vi "ACDC_Config.vi"(8 "error in (no error)":errorcluster, 9 "Input Config Array":T1[](array[typedef])=[0, 0, 0, 0, 0, 0, 0, 0, 0, 0, 0, 0, 0, 0, 0, 0, 0, 0, 0, 0, 0, 0, 0, 0, 0, 0, 0, 0, 0, 0, 0, 0] items=["AC Coupled", "DC Coupled", "IEPE AC Coupled"], 10 "Data Rate [S/s]":u32) -> (0 "error out":errorcluster)   [LabVIEW 2017, in "BOP_VibAPI_6.lvlib"]
uses:
  <vilib>/addons/InsightCM/Devices/Shared/Cms/Fpga/Acquisition/source/subVIs/VibAPI/BOP_VibAPI_6.lvlib
  <vilib>/LabVIEW Targets/FPGA/cRIO/shared/nicrio_ModuleControls/nicrio_cRIO-9232_ConfigModeRing.ctl
  <vilib>/rvi/eio/common/nirviEmuTemplatePropertySet_errors.vi
  <vilib>/eio/EIOPropertyNode/EIOPropertyNode.xnode
  <vilib>/LabVIEW Targets/FPGA/cRIO/shared/nicrio_ModuleControls/nicrio_cRIO-9232_DataRatesRing2.ctl
  <vilib>/rvi/eio/common/nirviEmuTemplatePropertyGet_errors.vi
  <vilib>/rvi/eio/common/nirviEmuTemplatePropertyGet_noerrors.vi
  <vilib>/rvi/eio/common/nirviEmuTemplatePropertySet_noerrors.vi
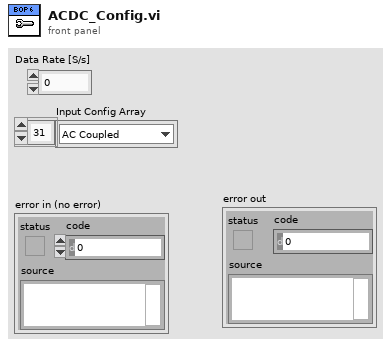
[diagram p1: front panel]
types:
  T1 = typedef "nicrio_cRIO-9232_ConfigModeRing.ctl" = u8
  T2 = typedef "nicrio_cRIO-9232_DataRatesRing2.ctl" = u8
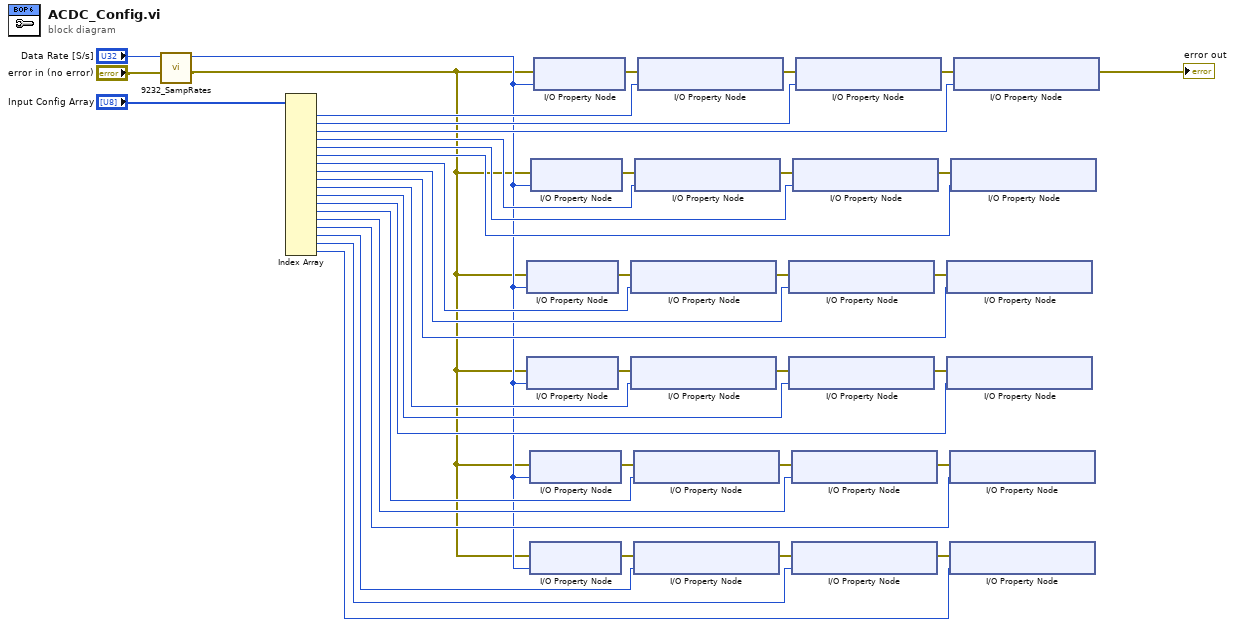
[diagram p0: block diagram]
diagram:
  n1 = call <vilib>:"9232_SampRates.vi"("error in (no error)"="error in (no error)", "Data Rate [S/s]"="Data Rate [S/s]") -> ("error out"=w3:errorcluster, "Data Rate"=w4:T2)  [unwired: 8 in]
  n2 = Index Array(array="Input Config Array") -> (element #1=w34:T1, element #2=w33:T1, element #3=w29:T1, element #4=w32:T1, element #5=w31:T1, element #6=w30:T1, element #7=w25:T1, element #8=w24:T1, element #9=w23:T1, element #10=w19:T1, element #11=w18:T1, element #12=w17:T1, element #13=w13:T1, element #14=w12:T1, element #15=w11:T1, element #16=w7:T1, element #17=w6:T1, element #18=w5:T1)  [unwired: 18 in]
  n3 = xnode "I/O Property Node"("error in"=w3, "Data Rate"=w4) -> ("error out"=w28:errorcluster)  [unwired: 1 in, 1 out]
  n4 = xnode "I/O Property Node"("error in"=w3, "Data Rate"=w4) -> ("error out"=w20:errorcluster)  [unwired: 1 in, 1 out]
  n5 = xnode "I/O Property Node"("error in"=w3, "Data Rate"=w4) -> ("error out"=w16:errorcluster)  [unwired: 1 in, 1 out]
  n6 = xnode "I/O Property Node"("error in"=w3, "Data Rate"=w4) -> ("error out"=w8:errorcluster)  [unwired: 1 in, 1 out]
  n7 = xnode "I/O Property Node"("error in"=w3, "Data Rate"=w4) -> ("error out"=w35:errorcluster)  [unwired: 1 in, 1 out]
  n8 = xnode "I/O Property Node"("error in"=w3, "Data Rate"=w4) -> ("error out"=w36:errorcluster)  [unwired: 1 in, 1 out]
  n9 = xnode "I/O Property Node"("error in"=w28, "Input Configuration"=w25) -> ("error out"=w27:errorcluster)  [unwired: 1 in, 1 out]
  n10 = xnode "I/O Property Node"("error in"=w20, "Input Configuration"=w19) -> ("error out"=w21:errorcluster)  [unwired: 1 in, 1 out]
  n11 = xnode "I/O Property Node"("error in"=w16, "Input Configuration"=w13) -> ("error out"=w15:errorcluster)  [unwired: 1 in, 1 out]
  n12 = xnode "I/O Property Node"("error in"=w8, "Input Configuration"=w7) -> ("error out"=w9:errorcluster)  [unwired: 1 in, 1 out]
  n13 = xnode "I/O Property Node"("error in"=w35, "Input Configuration"=w32) -> ("error out"=w39:errorcluster)  [unwired: 1 in, 1 out]
  n14 = xnode "I/O Property Node"("error in"=w36, "Input Configuration"=w34) -> ("error out"=w37:errorcluster)  [unwired: 1 in, 1 out]
  n15 = xnode "I/O Property Node"("error in"=w27, "Input Configuration"=w24) -> ("error out"=w26:errorcluster)  [unwired: 1 in, 1 out]
  n16 = xnode "I/O Property Node"("error in"=w21, "Input Configuration"=w18) -> ("error out"=w22:errorcluster)  [unwired: 1 in, 1 out]
  n17 = xnode "I/O Property Node"("error in"=w15, "Input Configuration"=w12) -> ("error out"=w14:errorcluster)  [unwired: 1 in, 1 out]
  n18 = xnode "I/O Property Node"("error in"=w9, "Input Configuration"=w6) -> ("error out"=w10:errorcluster)  [unwired: 1 in, 1 out]
  n19 = xnode "I/O Property Node"("error in"=w39, "Input Configuration"=w31) -> ("error out"=w40:errorcluster)  [unwired: 1 in, 1 out]
  n20 = xnode "I/O Property Node"("error in"=w37, "Input Configuration"=w33) -> ("error out"=w38:errorcluster)  [unwired: 1 in, 1 out]
  n21 = xnode "I/O Property Node"("error in"=w26, "Input Configuration"=w23) -> ()  [unwired: 1 in, 2 out]
  n22 = xnode "I/O Property Node"("error in"=w22, "Input Configuration"=w17) -> ()  [unwired: 1 in, 2 out]
  n23 = xnode "I/O Property Node"("error in"=w14, "Input Configuration"=w11) -> ()  [unwired: 1 in, 2 out]
  n24 = xnode "I/O Property Node"("error in"=w10, "Input Configuration"=w5) -> ()  [unwired: 1 in, 2 out]
  n25 = xnode "I/O Property Node"("error in"=w40, "Input Configuration"=w30) -> ()  [unwired: 1 in, 2 out]
  n26 = xnode "I/O Property Node"("error in"=w38, "Input Configuration"=w29) -> ("error out"=→"error out":errorcluster)  [unwired: 1 in, 1 out]
